vi "Test RoundTrip 2D Empty Array.vi"(8 "error in (no error)":errorcluster) -> (0 "error out":errorcluster)   [LabVIEW 2020]
uses:
  <vilib>/addons/_JKI Toolkits/Caraya/classes/Test/Test.lvclass
  <vilib>/addons/_JKI Toolkits/Caraya/classes/Assert/Assert.lvclass
  src/JKI JSON Serialization.lvlib
panel:
  out "JSON String":string
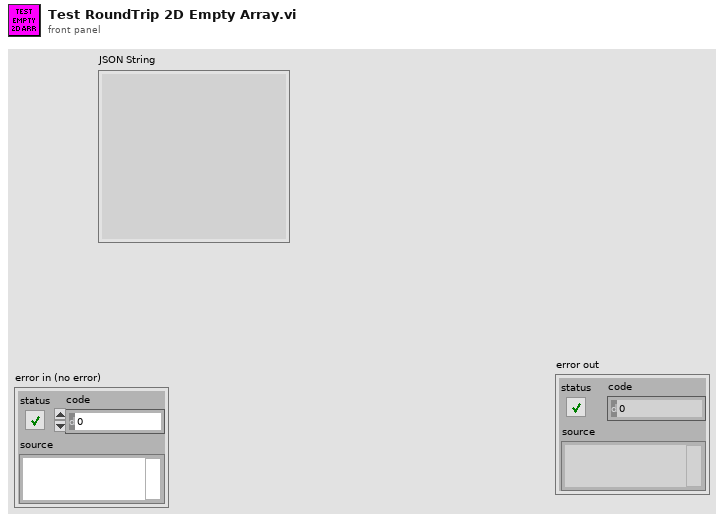
[diagram p1: front panel]
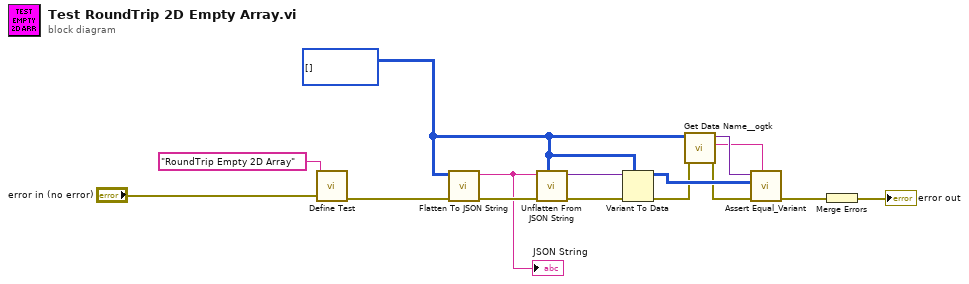
[diagram p0: block diagram]
diagram:
  w1 = i32[][] []
  n1 = call <vilib>:"Define Test.vi"("error in (no error)"="error in (no error)", "Label (VI Title)"="RoundTrip Empty 2D Array") -> ("error out"=w11:errorcluster)  [unwired: 9 in]
  n2 = call "Flatten To JSON String.vi"("error in (no error)"=w11, "Variant"=w1) -> ("error out"=w10:errorcluster, "JSON String"=w2:string)  [unwired: 8 in]
  "JSON String" <- w2
  n3 = call "Unflatten From JSON String.vi"("Type and Defaults"=w1, "error in (no error)"=w10, "JSON String"=w2) -> ("error out"=w7:errorcluster, "Variant"=w9:variant)  [unwired: 7 in]
  n4 = Variant To Data(error in=w7, type=w1, Variant=w9) -> (data=w8:i32[][], error out=w4:errorcluster)
  n5 = call <userlib>:"Get Data Name__ogtk.vi"("error in (no error)"=w4, "Data"=w1) -> ("error out"=w3:errorcluster, "Data Name"=w5:string, "Data dup"=w6:variant)  [unwired: 7 in]
  n6 = call <vilib>:"Assert Equal_Variant.vi"("Label"=w5, "error in (no error)"=w3, "Y"=w8, "X"=w6) -> ("error out"=w13:errorcluster)  [unwired: 7 in]
  n7 = Merge Errors(w13) -> (→"error out":errorcluster)
